vi "Available Registers FG.vi"(8 "error in (no error)":errorcluster, 11 "Item Ref":T3 format="%.0x") -> (0 "error out":errorcluster, 2 "Available Registers":T1[](array[typedef]) {"Data Type" format="%.0x"}, 3 "Item Ref out":T3=18446744073709551615 format="%.0x")   [LabVIEW 2016, in "FPGA Addon Shared.lvlib"]
uses:
  FPGA Addon Shared.lvlib
  <vilib>/NI Veristand/Custom Device API/Custom Device Item Ref.ctl
  Register Information.ctl
  Data Type.ctl
  <vilib>/rvi/Bitfile/nirviControlStructure.ctl
  <vilib>/rvi/Bitfile/nirviTypdefDescription.ctl
  <vilib>/rvi/Bitfile/nirviMechanicalAction.ctl
  <vilib>/rvi/Bitfile/nirviSubControlStructure.ctl
  <vilib>/rvi/Bitfile/nirviClusterElementControl.ctl
  RM Client API/get fgpa resources.vi
  RM Client API/find Relative VS Ref.vi
  <vilib>/NI Veristand/Custom Device API/NI VeriStand - Get Item Data.vi
  <vilib>/NI VeriStand/Custom Device API/Custom Device API.lvlib
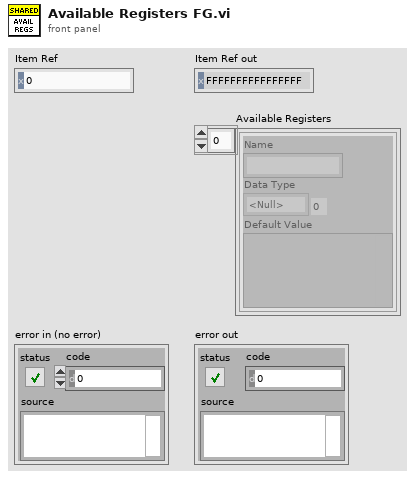
[diagram p1: front panel]
types:
  T1 = typedef "FPGA Addon Shared.lvlib/Register Information.ctl" = cluster{"Name":string, "Data Type":T2, "Default Value":variant}
  T2 = typedef "FPGA Addon Shared.lvlib/Data Type.ctl" = enum8{"<Null>", "I8", "I16", "I32", "I64", "U8", "U16", "U32", "U64", "SGL", "Boolean", "Analog PWM In Settings", "Analog PWM In", "Digital PWM In Settings", "Digital PWM In", "Digital PWM Out", "Sine Out", "FXP+/-24.5", "FXP+/-16.5", "FXP+/-32.8", "FXP+/-64.32", "FXP+/-16.7", "FXP+/-20.5"}
  T3 = typedef "Custom Device API.lvlib/Custom Device Item Ref.ctl" = u64
  T4 = typedef "nirviControlStructure.ctl" = cluster{"Name":string, "Hidden":bool, "Indicator":bool, "Flattened Type":string, "Grouping":cluster{"Grouped":bool, "Member Names":string[], "Member IDs":u32[]}, "Address":u32, "Size":u32, "Class":u32, "Internal":bool, "Typedef":T5, "ID":u32, "Bidirectional":bool, "Synchronous":bool, "Mechanical Action":T6, "Sub Controls":T7[], "Access May Timeout":bool, "Register Node":bool}
  T5 = typedef "nirviTypdefDescription.ctl" = cluster{"Typedef":bool, "Path":path}
  T6 = typedef "nirviMechanicalAction.ctl" = enum8{"Switch When Pressed", "Switch When Released", "Switch Until Released", "Latch When Pressed", "Latch When Released", "Latch Until Released"}
  T7 = typedef "nirviSubControlStructure.ctl" = cluster{"Name":string, "flattened Type":string, "Cluster Information":T8, "Typedef":T5}
  T8 = typedef "nirviClusterElementControl.ctl" = cluster{"Name Hierarchy":string[], "Item Order":u32[]}
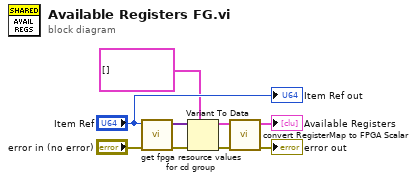
[diagram p0: block diagram]
diagram:
  n1 = call "get fpga resource values for cd group.vi"("error in (no error)"="error in (no error)", "Item Ref"="Item Ref") -> ("error out"=w1:errorcluster, "fpga resources"=w5:variant[])  [unwired: 8 in]
  n2 = Variant To Data(error in=w1, type=T4[] [] ("RegisterMap"), Variant=w5) -> (data=w3:T4[], error out=w2:errorcluster)
  n3 = call "convert RegisterMap to FPGA Scalar.vi"("error in"=w2, "RegisterMap"=w3) -> ("error out"=→"error out":errorcluster, "FPGA Scalar"=→"Available Registers":T1[])  [unwired: 8 in]
  "Item Ref out" <- "Item Ref"
